vi "16-1.vi"() -> ()   [LabVIEW 2019, in "16.lvlib"]
uses:
  16.lvlib
panel:
  out "Remaining BITS":bool[](array[boolean])
  out "Packet":T1
  out "Version Sum":u32
  in  "Sample Index":i32
  in  "Sample":bool=TRUE
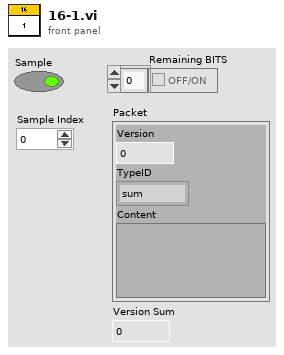
[diagram p1: front panel]
types:
  T1 = cluster{"Version":u32, "TypeID":enum16{"sum", "product", "minimum", "maximum", "literal", "greater than", "less than", "equal to"}, "Content":variant}
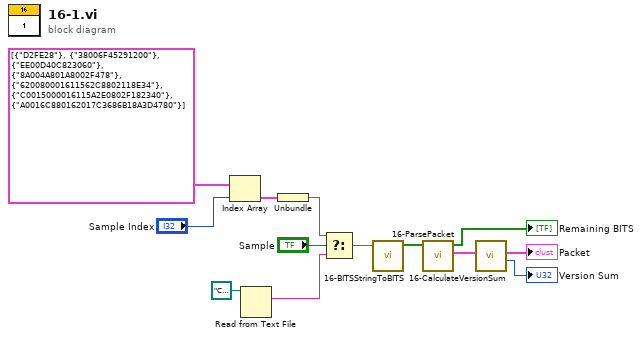
[diagram p0: block diagram]
diagram:
  n1 = Index Array(array=cluster{string}[] [{"D2FE28"}, {"38006F45291200"}, {"EE00D40C823060"}, {"8A004A801A8002F478"}, {"620080001611562C8802118E34"}, {"C0015000016115A2E0802F182340"}, {"A0016C880162017C3686B18A3D4780"}], index="Sample Index") -> (element=w11:cluster{string})
  n2 = Read from Text File(file (use dialog)=path "C:/Users/craig.walker/Documents/GitHub/lv2019-Advent-of-Code-2021/16/input.txt") -> (text=w7:string)  [unwired: 3 in, 3 out]
  n3 = Unbundle(w11) -> (w8:string)
  n4 = Select(t=w8, s="Sample", f=w7) -> (s? t:f=w9:string)
  n5 = call "16-BITSStringToBITS.vi"("BITS String"=w9) -> ("BITS out"=w13:bool[])  [unwired: 10 in]
  n6 = call "16-ParsePacket.vi"("BITS in"=w13) -> ("Packet"=w4:T1, "BITS out"=→"Remaining BITS":bool[])  [unwired: 9 in]
  n7 = call "16-CalculateVersionSum.vi"("Packet in"=w4) -> ("Version Sum"=→"Version Sum":u32, "Packet out"=→"Packet":T1)  [unwired: 9 in]
